vi "Configure Modulation Low Level (Source).vi"(8 "error in (no error)":errorcluster, 9 "Source (Internal)":enum16{"Internal", "External"}(ring), 10 "Modulation (AM)":enum16{"AM", "FM", "PM", "FSK", "PWM"}(ring), 11 "VISA resource name":refnum<visa-resource-name>) -> (0 "error out":errorcluster, 3 "VISA resource name out":refnum<visa-resource-name>)   [LabVIEW 2017, in "Keithley 3390.lvlib"]
uses:
  Keithley 3390.lvlib
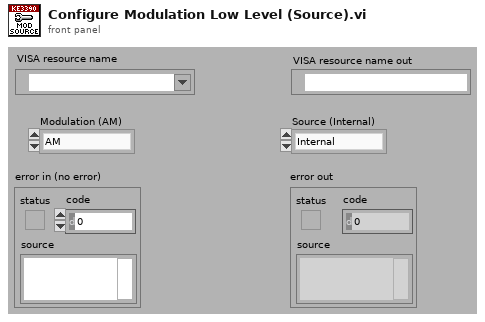
[diagram p1: front panel]
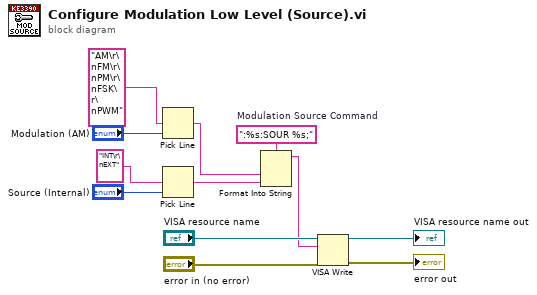
[diagram p0: block diagram]
diagram:
  w6 = ":%s:SOUR %s;"  # Modulation Source Command
  n1 = Pick Line(multi-line string="AM\r\nFM\r\nPM\r\nFSK\r\nPWM" ("options"), line index="Modulation (AM)") -> (output string=w5:string)  [unwired: 1 in]
  n2 = Pick Line(multi-line string="INT\r\nEXT" ("options"), line index="Source (Internal)") -> (output string=w4:string)  [unwired: 1 in]
  n3 = Format Into String(format string=w6, w5, w4) -> (resulting string=w3:string)  [unwired: 2 in, 1 out]
  n4 = VISA Write(VISA resource name="VISA resource name", write buffer=w3, error in (no error)="error in (no error)") -> (VISA resource name out=→"VISA resource name out":refnum<visa-resource-name>, error out=→"error out":errorcluster)  [unwired: 1 out]
